vi "LWXPS_CIEHeaderGet.vi"(0 "XPS Reference IN":refnum<k24>, 7 "CIE Board Index":i32, 11 "LabVIEW error IN":errorcluster) -> (4 "XPS Reference OUT":refnum<k24>, 6 "Returned error code":i32, 8 "Header String":string, 10 "XPS Error String":string, 15 "LabVIEW error OUT":errorcluster)   [LabVIEW 2014]
uses:
  D:/XPSQ8_LabView_Library/Development/Source/Dll/Newport.XPS.CommandInterface.dll
  Dll/Newport.XPS.CommandInterface.dll
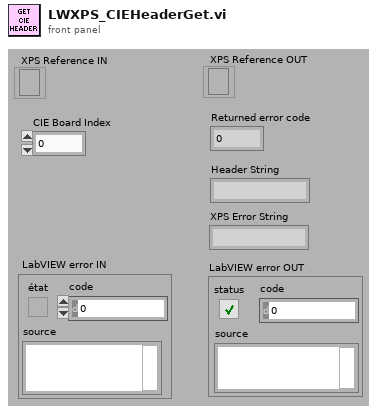
[diagram p1: front panel]
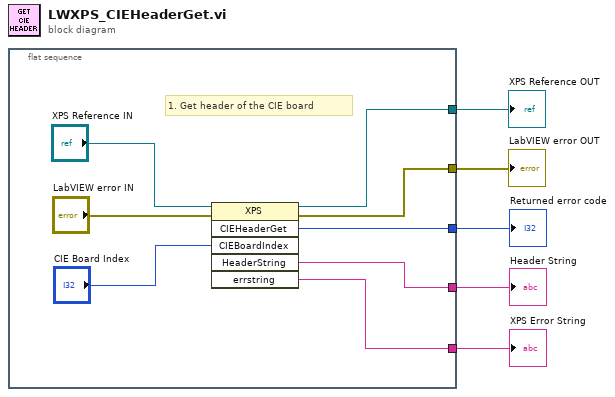
[diagram p0: block diagram]
diagram:
  n1 = flat-sequence {
    tunnel: [w11] -> w5
    tunnel: [w10] -> w4
    tunnel: [w9] -> w3
    tunnel: [w8] -> w2
    tunnel: [w7] -> w1
    frame #0 {
      # "1. Get header of the CIE board"
      n2 = invoke class="XPS" method="CIEHeaderGet"(reference="XPS Reference IN", error in="LabVIEW error IN", "CIEBoardIndex"="CIE Board Index") -> (reference out=w11:refnum<k24>, error out=w10:errorcluster, "CIEHeaderGet"=w7:i32, "HeaderString"=w8:string, "errstring"=w9:string)  [unwired: 3 in, 1 out]
    }
  }
  "XPS Reference OUT" <- w5
  "LabVIEW error OUT" <- w4
  "XPS Error String" <- w3
  "Header String" <- w2
  "Returned error code" <- w1
